vi "Init.vi"(1 "GraphButtons":refnum<vi>, 5 "error in (no error)":errorcluster) -> (15 "Event":refnum<user-event>, 19 "error out":errorcluster)   [LabVIEW 2016, in "UmlEditor.lvclass"]
uses:
  <resource>/Framework/Providers/Open_GDS/UML/UmlEditor_class/UmlEditor.lvclass
  <resource>/Framework/Providers/Open_GDS/UML/UmlEditor_class/EventData.ctl
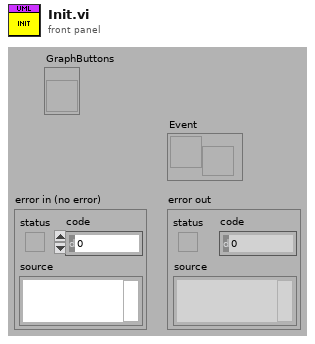
[diagram p1: front panel]
types:
  T1 = typedef "UmlEditor.lvclass/EventData.ctl" = cluster{"Action":string, "Data":string}
  T2 = typedef "UmlEditor.lvclass/ObjectAttributes.ctl" = cluster{"ListeningQueueIn":refnum<queue>, "Event":refnum<user-event>, "UseProjectFolderAsBasePath":bool, "TypeSyncOption":bool, "Attr":string[], "ToolTip":cluster{"ToolTipOpen":bool, "LastToolTip":i32}, "ClassesToIgnore":string[], "UndoSize":i32, "OpenLastSavedFileWhenStarting":bool, "SyncOption":T3, "SyncTime(s)":i32, "Params":cluster{"IniParams":T4, "Value":string}[], "GraphButtons":refnum<vi>}
  T3 = typedef "UMLEditor_SyncOptions.ctl" = cluster{"IgnoreInstrLib":bool, "IgnoreUserLib":bool, "IgnoreViLib":bool}
  T4 = typedef "UmlEditor.lvclass/IniParamsType.ctl" = enum16{"I have problem with UML stability on my computer"}
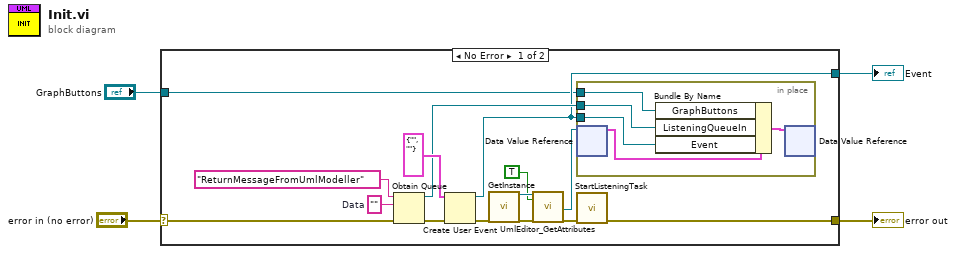
[diagram p0: block diagram]
diagram:
  n1 = case shown="No Error" "error in (no error)" {
    selector: "error in (no error)" -> [w15 w25]
    tunnel: [w16 w25] -> w3
    tunnel: [w6 _] -> w2
    tunnel: "GraphButtons" -> [w5 _]
    frame No Error {
      w13 = ""  # Data
      n2 = Obtain Queue(name (unnamed)="ReturnMessageFromUmlModeller", element data type=w13, error in (no error)=w15) -> (queue out=w7:refnum<queue>, error out=w12:errorcluster)  [unwired: 2 in, 1 out]
      n3 = Create User Event(user event datatype=T1 {"Action"="", "Data"=""} ("EventData"), error in=w12) -> (user event=w6:refnum<user-event>, error out=w10:errorcluster)
      n4 = call <resource>:"GetInstance.vi"("error in (no error)"=w10) -> ("reference out"=w19:refnum<class "UmlEditor.lvclass">, "error out"=w18:errorcluster)  [unwired: 17 out]
      n5 = call <resource>:"UmlEditor_GetAttributes.vi"("reference in"=w19, "OnlyGetDvrReference(False)"=TRUE, "error in (no error)"=w18) -> ("DataRef"=w8:refnum<data-value>, "error out"=w17:errorcluster)  [unwired: 13 in, 2 out]
      n6 = in-place {
        in-place-border: w7 -> [w23]
        in-place-border: w6 -> [w22]
        in-place-border: w5 -> [w20]
        n7 = in-place-dvr #1(w8) -> (w24:T2)  [unwired: 1 out]
        n8 = Bundle By Name(cluster=w24, "GraphButtons"=w20, "ListeningQueueIn"=w23, "Event"=w22) -> (w21:T2)
        n9 = in-place-dvr #1(w21) -> ()  [unwired: 2 out]
      }
      n10 = call <resource>:"StartListeningTask.vi"("error in (no error)"=w17) -> ("error out"=w16:errorcluster)  [unwired: 10 out]
    }
    frame Error {
    }
  }
  "error out" <- w3
  "Event" <- w2
